vi "checkin.vi"(8 "error in (no error)":errorcluster, 11 "GenericScanMode in":refnum<class "GenericImagingMode.lvclass">) -> (0 "error out":errorcluster, 3 "GenericScanMode out":refnum<class "GenericImagingMode.lvclass">)   [LabVIEW 2010, in "GenericImagingMode.lvclass"]
uses:
  GenericImagingMode.lvclass
  common/classes/GenericToplevelComponent/GenericToplevelComponent/GenericToplevelComponent.lvclass
  class_data.vi
  common/classes/ErrorController/ErrorController/class_data.vi
  common/classes/GenericComponent/GenericComponent/GenericComponent.lvclass
  common/classes/ErrorController/ErrorController/ErrorController.lvclass
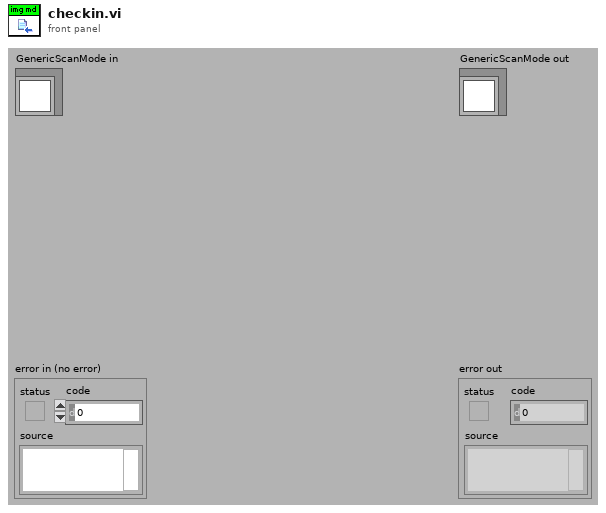
[diagram p1: front panel]
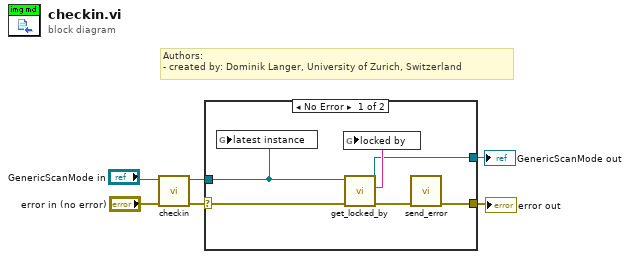
[diagram p0: block diagram]
diagram:
  # "Authors: \n- created by: Dominik Langer, University of Zurich, Switzerland"
  n1 = call-parent "checkin.vi"("error in (no error)"="error in (no error)", "GenericPlugin in"="GenericScanMode in") -> ("error out"=w3:errorcluster, "GenericPlugin out"=w1:refnum<class "GenericImagingMode.lvclass">)  [unwired: 8 in]
  n2 = case shown="No Error" w3 {
    selector: w3 -> [w7 w14]
    tunnel: [w9 w14] -> w5
    tunnel: [w11 w13] -> w6
    tunnel: w1 -> [w8 w13]
    frame No Error {
      n3 = global write "class_data.vi" "latest instance"(w8) -> ()
      n4 = call "get_locked_by.vi"("error in (no error)"=w7, "GenericPlugin.lvclass in"=w8) -> ("error out"=w10:errorcluster, "locked by"=w12:string, "GenericPlugin.lvclass out"=w11:refnum<class "GenericImagingMode.lvclass">)  [unwired: 7 out]
      n5 = global write "class_data.vi" "locked by"(w12) -> ()
      n6 = call "send_error.vi"("error in (no error)"=w10) -> ("error out"=w9:errorcluster)  [unwired: 10 in]
    }
    frame Error {
    }
  }
  "error out" <- w5
  "GenericScanMode out" <- w6
